vi "Read Voltage Actual.vi"   [LabVIEW 2023, in "Cycler.lvclass"]
uses:
  Cycler.lvclass
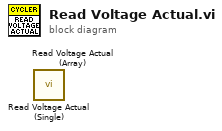
[diagram p0: block diagram]
diagram:
  n1 = call "Read Voltage Actual (Single).vi"() -> ()  [unwired: 8 in, 4 out]
  n2 = call "Read Voltage Actual (Array).vi"() -> ()  [unwired: 8 in, 4 out]
